vi "finalize initialization.vi"(8 "error in":errorcluster, 10 "configuration in":refnum<class "fixed channel configuration.lvclass">, 11 "Temperature Chamber Model runtime in":refnum<class "Temperature Chamber Model runtime.lvclass">) -> (0 "error out":errorcluster, 3 "Temperature Chamber Model runtime out":refnum<class "Temperature Chamber Model runtime.lvclass">)   [LabVIEW 2013, in "Temperature Chamber Model runtime.lvclass"]
uses:
  Temperature Chamber Model runtime.lvclass
  <vilib>/NI/Tag Bus Data Framework/fixed module parent/module/configuration/fixed channel configuration.lvclass
  configuration/Temperature Chamber Model configuration.lvclass
  model state.ctl
  Temperature Chamber Model runtime.lvclass/Temperature Chamber Model runtime.ctl
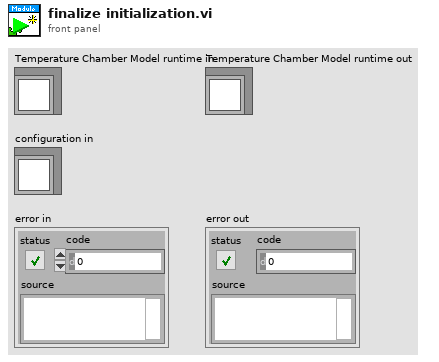
[diagram p1: front panel]
types:
  T1 = typedef "Temperature Chamber Model runtime.lvclass/model state.ctl" = cluster{"Previous Temperature":dbl, "Previous Tick Count":u32, "Just Initialized?":bool}
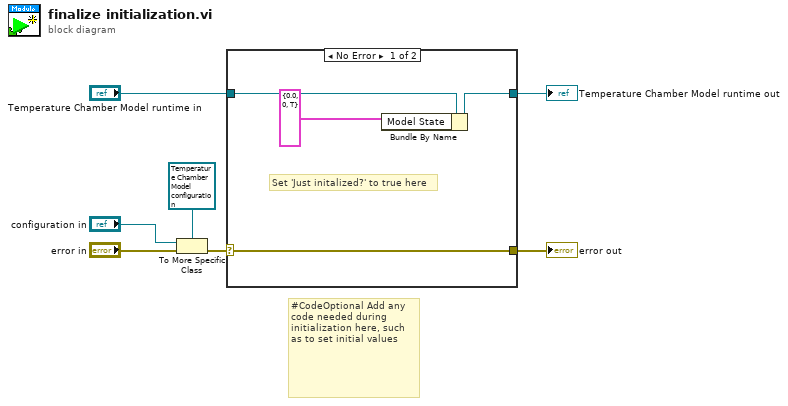
[diagram p0: block diagram]
diagram:
  # "#CodeOptional Add any code needed during initialization here, such as to set initial values"
  n1 = To More Specific Class(target class=refnum<class "Temperature Chamber Model configuration.lvclass"> refnum ("user module configuration"), reference="configuration in", error in="error in") -> (error out=w4:errorcluster)  [unwired: 1 out]
  n2 = case shown="No Error" w4 {
    selector: w4 -> [w11 w12]
    tunnel: [w8 w13] -> w3
    tunnel: "Temperature Chamber Model runtime in" -> [w10 w13]
    tunnel: [w11 w12] -> w1
    frame No Error {
      # "Set 'Just initalized?' to true here"
      n3 = Bundle By Name(cluster=w10, "Model State"=T1 {"Previous Temperature"=0.0, "Previous Tick Count"=0, "Just Initialized?"=TRUE}) -> (w8:refnum<class "Temperature Chamber Model runtime.lvclass">)
    }
    frame Error {
    }
  }
  "error out" <- w1
  "Temperature Chamber Model runtime out" <- w3
